vi "acqChanData.vi"(8 "errorIn":errorcluster, 10 "chanName":string, 11 "ACQ":T2) -> (0 "error out":errorcluster caption="errorOut", 2 "channel":T1, 3 "shotNum":string)   [LabVIEW 2017]
uses:
  models/ACQ.ctl
  models/Header.ctl
  models/ACQ_channel.ctl
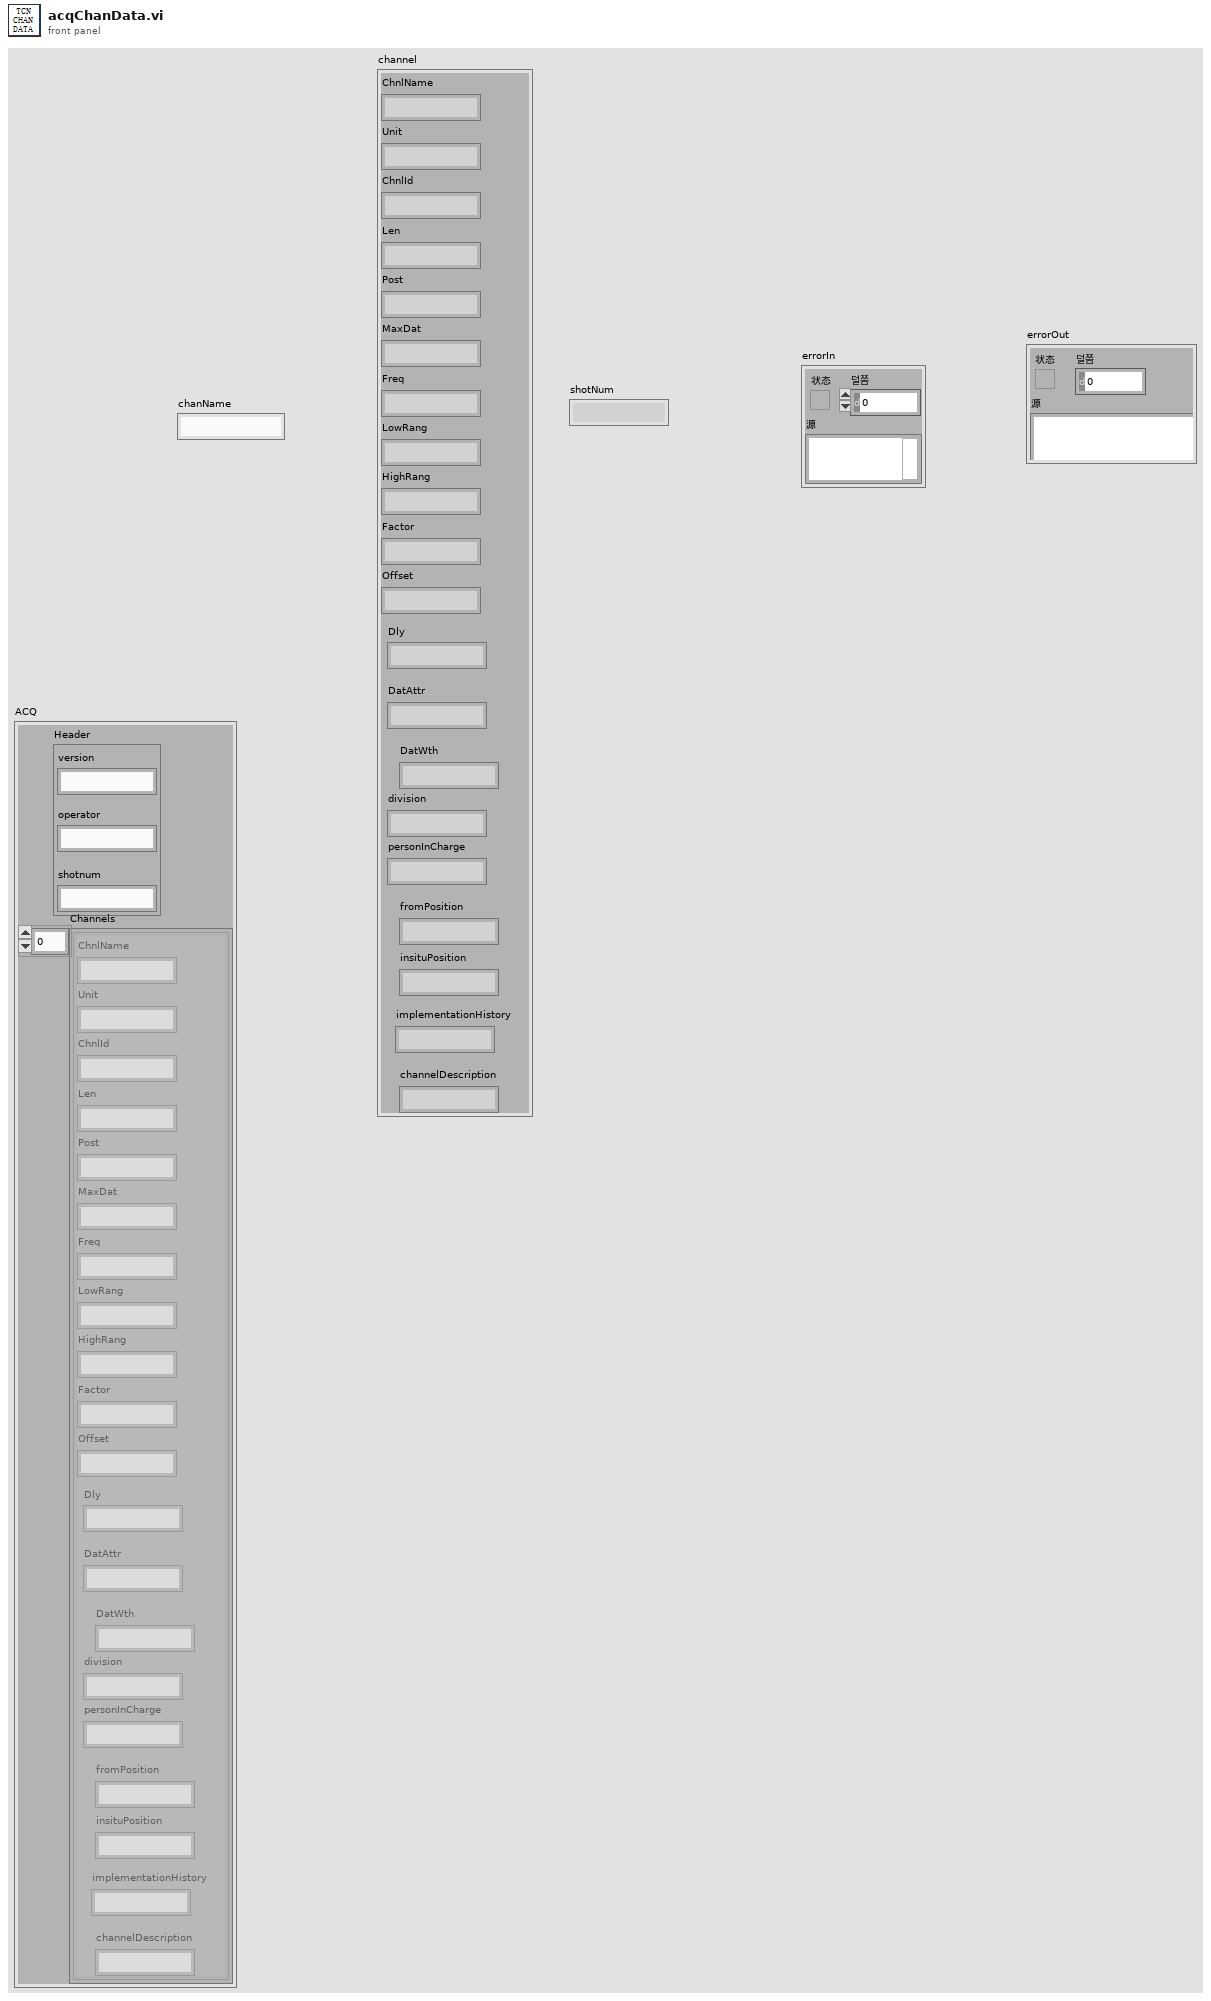
[diagram p1: front panel]
types:
  T1 = typedef "ACQ_channel.ctl" = cluster{"ChnlName":string, "Unit":string, "ChnlId":string, "Len":string, "Post":string, "MaxDat":string, "Freq":string, "LowRang":string, "HighRang":string, "Factor":string, "Offset":string, "Dly":string, "DatAttr":string, "DatWth":string, "division":string, "personInCharge":string, "fromPosition":string, "insituPosition":string, "implementationHistory":string, "channelDescription":string}
  T2 = typedef "ACQ.ctl" = cluster{"Header":T3, "Channels":T1[]}
  T3 = typedef "Header.ctl" = cluster{"version":string, "operator":string, "shotnum":string}
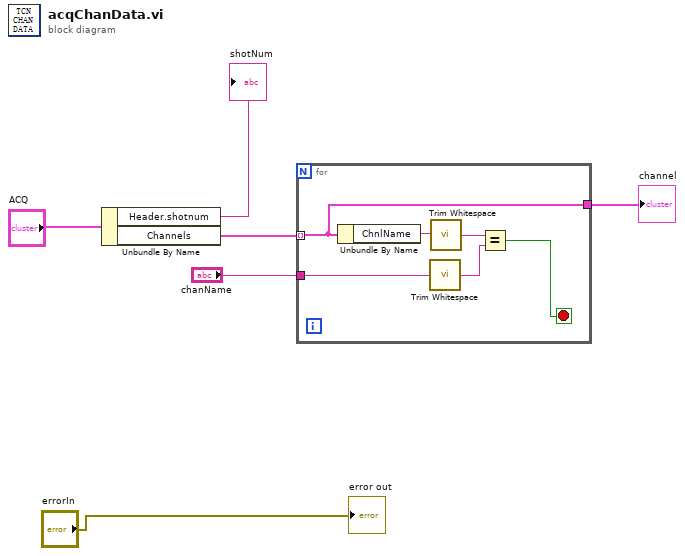
[diagram p0: block diagram]
diagram:
  n1 = Unbundle By Name("ACQ") -> ("Header.shotnum"=→"shotNum":string, "Channels"=w6:T1[])
  n2 = for {
    tunnel: w6 -> [w7] mode=indexing
    tunnel: "chanName" -> [w11]
    tunnel: [w7] -> w2
    stop <- w8 stop-if-true
    n3 = Unbundle By Name(w7) -> ("ChnlName"=w12:string)
    n4 = call <vilib>:"Trim Whitespace.vi"("string"=w11) -> ("trimmed string"=w9:string)  [unwired: 1 in]
    n5 = call <vilib>:"Trim Whitespace.vi"("string"=w12) -> ("trimmed string"=w10:string)  [unwired: 1 in]
    n6 = Equal?(x=w10, y=w9) -> (x = y?=w8:bool)
  }
  "channel" <- w2
  "error out" <- "errorIn"
